vi "Event-Activate.vi"(8 "error in (no error)":errorcluster, 10 "Data ref. in":refnum<data-value>, 11 "UI ref. in":refnum<data-value>) -> (0 "error out":errorcluster, 2 "Data ref.":refnum<data-value>, 3 "UI ref.":refnum<data-value>)   [LabVIEW 2013, in "CameraVision.lvlib" / "CV-UI.lvclass"]
uses:
  CV-UI.lvclass
  Main/CV-Main.lvclass
  Main/Main-actions.ctl
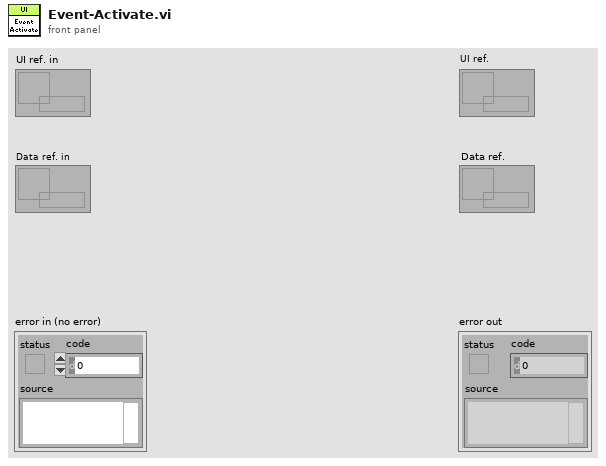
[diagram p1: front panel]
types:
  T1 = typedef "CameraVision.lvlib/CV-Main.lvclass/Main-actions.ctl" = enum16{"Idle", "Initialize", "Load defaults", "Update settings", "Check settings", "Save settings", "Save settings with dialog", "Load settings", "Load data", "Activate", "Start", "Wait for start signal", "Acquire & process", "Iterate", "Stop", "Refresh display", "Refresh status", "View camera settings", "View grabber settings", "Exit"}
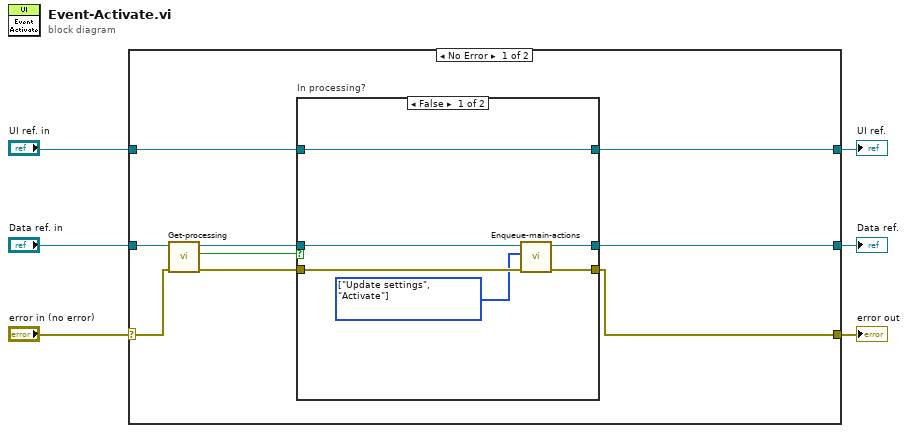
[diagram p0: block diagram]
diagram:
  n1 = case shown="No Error" "error in (no error)" {
    selector: "error in (no error)" -> [w7 w27]
    tunnel: [w8 w27] -> w5
    tunnel: [w12 w26] -> w3
    tunnel: "UI ref. in" -> [w10 w26]
    tunnel: "Data ref. in" -> [w15 w25]
    tunnel: [w11 w25] -> w1
    frame No Error {
      n2 = call "Get-processing.vi"("error in (no error)"=w7, "Data ref. in"=w15) -> ("error out"=w9:errorcluster, "Processing?"=w13:bool, "Data ref."=w14:refnum<data-value>)  [unwired: 7 in]
      n3 = case "In processing?" shown="False" w13 {
        tunnel: w10 -> [w20 w24]
        tunnel: w14 -> [w21 w23]
        tunnel: [w20 w24] -> w12
        tunnel: [w19 w23] -> w11
        tunnel: w9 -> [w17 w22]
        tunnel: [w18 w22] -> w8
        frame False {
          w16 = T1[] [enum."Update settings", enum."Activate"] items=["Idle", "Initialize", "Load defaults", "Update settings", "Check settings", "Save settings", "Save settings with dialog", "Load settings", "Load data", "Activate", "Start", "Wait for start signal", "Acquire & process", "Iterate", "Stop", "Refresh display", "Refresh status", "View camera settings", "View grabber settings", "Exit"] ("State array")
          n4 = call "Enqueue-main-actions.vi"("error in (no error)"=w17, "State array"=w16, "Data ref. in"=w21) -> ("error out"=w18:errorcluster, "Data ref."=w19:refnum<data-value>)  [unwired: 6 in, 1 out]
        }
        frame True {
        }
      }
    }
    frame Error {
    }
  }
  "error out" <- w5
  "Data ref." <- w1
  "UI ref." <- w3
